vi "Config.vi"(8 "error in (no error)":errorcluster, 10 "Digital Configuration Parameters":T1) -> (0 "error out":errorcluster, 3 "TCP 380 out":refnum<class "TCP 380.lvclass">)   [LabVIEW 2021, in "TCP 380.lvclass"]
uses:
  TCP 380.lvclass
  <vilib>/NathanCo/Digital-Tasks/Utilities/Digital Configuration Parameters.ctl
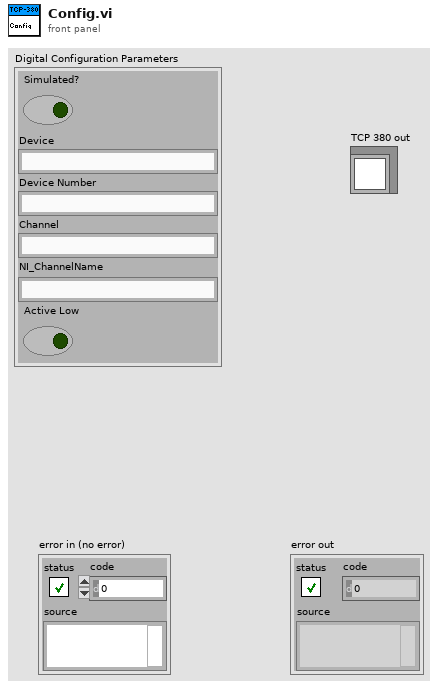
[diagram p1: front panel]
types:
  T1 = typedef "Digital Configuration Parameters.ctl" = cluster{"Simulated?":bool, "Device":string, "Device Number":string, "Channel":string, "NI_ChannelName":string, "Active Low":bool}
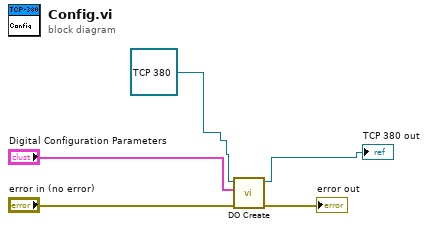
[diagram p0: block diagram]
diagram:
  n1 = call "DO Create.vi"("error in (no error)"="error in (no error)", "Digital Configuration Parameters"="Digital Configuration Parameters", "TCP 380 in"=refnum<class "TCP 380.lvclass"> refnum ("TCP 380.lvclass")) -> ("error out"=→"error out":errorcluster, "TCP 380 out"=→"TCP 380 out":refnum<class "TCP 380.lvclass">)  [unwired: 7 in]
